vi "img_make_cam2.vi"() -> ()   [LabVIEW 2016]
uses:
  <vilib>/userdefined/High Color/IMAQdx.ctl
  <vilib>/Utility/file.llb/Write Delimited Spreadsheet (I64).vi
  <vilib>/vision/NI_Vision_Development_Module.lvlib
  <vilib>/vision/driver/NI_Vision_Acquisition_Software.lvlib
panel:
  in  "Session In":T1="cam1"
  out "Image Pixels (U8)":u8[][](array[numeric])
  in  "save":bool
  out "img_min_val":u8
  out "img_max_val":u8
  in  "Color Plane":i32(ring)=1 items=["Red", "Green", "Blue", "Hue", "Saturation", "Luminance", "Value", "Intensity"]
  out "error out":errorcluster
  out "Image_ori":T2(plugin-control)
  in  "Optional Rectangle":i32[](array[numeric])=[508, 77, 838, 531]
  in  "fname":string="lego"
  out "size_check":i32[](array[numeric])=[28, 28]
  in  "fpath_jpg":path=path "C:/Users/NB-SH-001/Documents/Python Scripts/data/img_face/01_surprise/surprise_img"
  in  "fpath_txt":path=path "C:/Users/NB-SH-001/Documents/Python Scripts/data/img_face/01_surprise/surprise_txt"
  in  "X Resolution":i32=28
  in  "Y Resolution":i32=28
  out "count":i32=91
  in  "정지":bool
  out "Image_resample":T2(plugin-control)
  # "Image file maker"
  # "28"
  # "28"
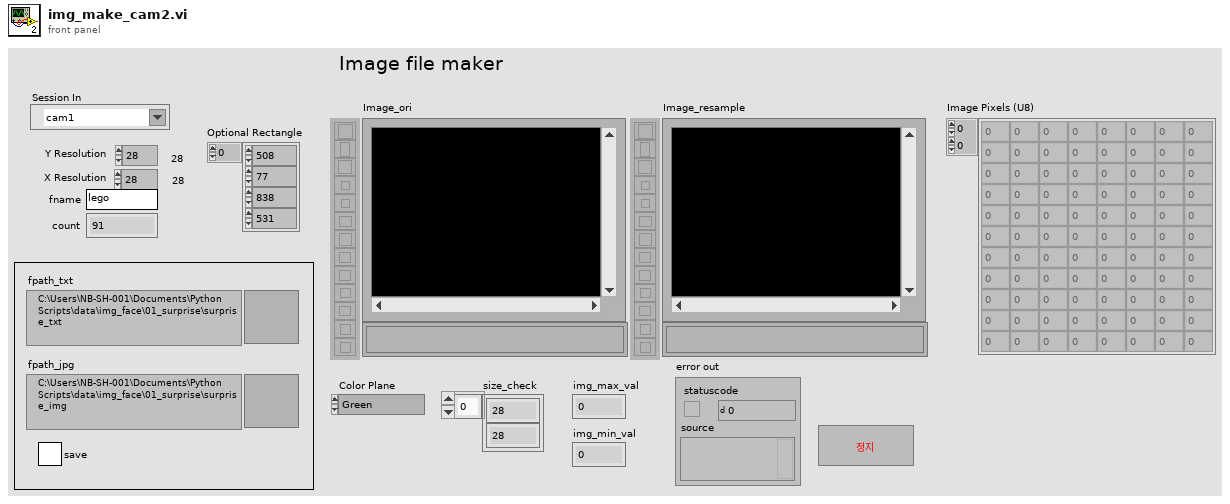
[diagram p1: front panel]
types:
  T1 = typedef "IMAQdx.ctl" = refnum<k21>
  T2 = typedef "IMAQ Image.ctl" = refnum<image>
  T3 = typedef "Image Type" = u32
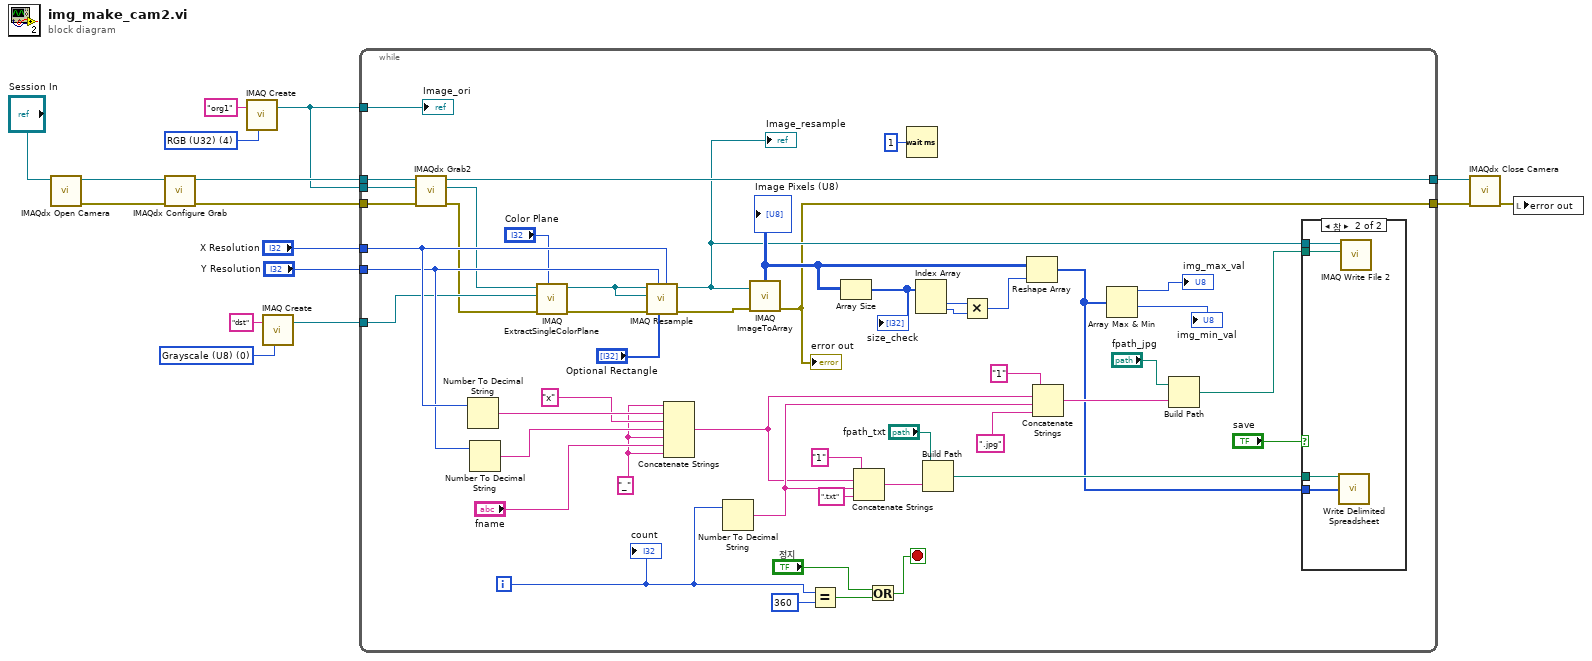
[diagram p0: block diagram]
diagram:
  w9 = T3 0 items=["Grayscale (U8)", "Grayscale (I16)", "Grayscale (SGL)", "Complex (CSG)", "RGB (U32)", "HSL (U32)", "RGB (U64)", "Grayscale (U16)"] ("Image Type")
  w15 = T3 4 items=["Grayscale (U8)", "Grayscale (I16)", "Grayscale (SGL)", "Complex (CSG)", "RGB (U32)", "HSL (U32)", "RGB (U64)", "Grayscale (U16)"] ("Image Type")
  n1 = call <vilib>:"IMAQdx Open Camera.vi"("Session In"="Session In") -> ("error out"=w11:errorcluster, "Session Out"=w12:T1)  [unwired: 9 in]
  n2 = call <vilib>:"IMAQdx Configure Grab.vi"("error in"=w11, "Session In"=w12) -> ("error out"=w7:errorcluster, "Session Out"=w6:T1)  [unwired: 8 in]
  n3 = call "IMAQ Create"("Image Name"="org1", "Image Type"=w15) -> ("New Image"=w3:T2)  [unwired: 3 in, 1 out]
  n4 = call "IMAQ Create"("Image Name"="dst", "Image Type"=w9) -> ("New Image"=w5:T2)  [unwired: 3 in, 1 out]
  n5 = while {
    tunnel: "X Resolution" -> [w34]
    tunnel: "Y Resolution" -> [w33]
    tunnel: w7 -> [w38]
    tunnel: w6 -> [w37]
    tunnel: w3 -> [w35]
    tunnel: w5 -> [w27]
    tunnel: [w32] -> w4
    tunnel: w3 -> [w29]
    tunnel: [w17] -> w2
    i -> [w57]
    stop <- w61 stop-if-true
    w40 = "_" ("문자열")
    n6 = call <vilib>:"IMAQdx Grab2.vi"("error in"=w38, "Image In"=w35, "Session In"=w37) -> ("error out"=w18:errorcluster, "Image Out"=w28:T2, "Session Out"=w32:T1)  [unwired: 5 in, 1 out]
    n7 = Number To Decimal String(number=w34) -> (decimal integer string=w44:string)  [unwired: 1 in]
    n8 = Number To Decimal String(number=w33) -> (decimal integer string=w42:string)  [unwired: 1 in]
    n9 = call "IMAQ ExtractSingleColorPlane"("Color Plane"="Color Plane", "error in (no error)"=w18, "Image Dst"=w27, "Image Src"=w28) -> ("error out"=w26:errorcluster, "Image Dst Out"=w30:T2)  [unwired: 6 in]
    n10 = call "IMAQ Resample"("X Resolution"=w34, "Optional Rectangle"="Optional Rectangle", "Y Resolution"=w33, "error in (no error)"=w26, "Image Dst"=w30, "Image Src"=w30) -> ("error out"=w22:errorcluster, "Image Dst Out"=w31:T2)  [unwired: 4 in]
    "Image_resample" <- w31
    n11 = Concatenate Strings(w40, w44, "x" ("문자열"), w42, w40, "fname", w40) -> (w39:string)
    n12 = Number To Decimal String(number=w57) -> (decimal integer string=w48:string)  [unwired: 1 in]
    n13 = call "IMAQ ImageToArray"("error in (no error)"=w22, "Image"=w31) -> ("error out"=w17:errorcluster, "Image Pixels (U8)"=w45:u8[][])  [unwired: 2 in, 3 out]
    "error out" <- w17
    "Image Pixels (U8)" <- w45
    n14 = Equal?(x=w57, y=360) -> (x = y?=w63:bool)
    n15 = Array Size(array=w45) -> (size(s)=w54:i32[])
    "size_check" <- w54
    n16 = Concatenate Strings("1" ("문자열"), w39, w48, ".txt" ("문자열")) -> (w59:string)
    n17 = Or(x="정지", y=w63) -> (x .or. y?=w61:bool)
    n18 = Wait (ms)(milliseconds to wait=u32 1 ("대기 시간 (ms)")) -> ()  [unwired: 1 out]
    n19 = Index Array(array=w54) -> (element #1=w52:i32, element #2=w53:i32)  [unwired: 2 in]
    n20 = Build Path(base path="fpath_txt", name or relative path=w59) -> (appended path=w21:path)
    n21 = Multiply(x=w52, y=w53) -> (x*y=w55:i32)
    n22 = Reshape Array(w45, w55) -> (w20:u8[])
    n23 = Concatenate Strings("1" ("문자열"), w39, w48, ".jpg" ("문자열")) -> (w50:string)
    n24 = Array Max & Min(array=w20) -> (max value=→"img_max_val":u8, min value=→"img_min_val":u8)  [unwired: 2 out]
    n25 = Build Path(base path="fpath_jpg", name or relative path=w50) -> (appended path=w46:path)
    n26 = case shown="참" "save" {
      tunnel: w46 -> [_ w69]
      tunnel: w31 -> [_ w68]
      tunnel: w21 -> [_ w67]
      tunnel: w20 -> [_ w66]
      frame False {
      }
      frame True {
        n27 = call-poly <vilib>:"Write Delimited Spreadsheet.vi"("file path (dialog if empty)"=w67, "1D data"=w66) -> ()  [unwired: 12 in, 2 out]
        n28 = call-poly "IMAQ Write File 2"("File Path"=w69, "Image"=w68) -> ()  [unwired: 8 in, 2 out]
      }
    }
    "count" <- w57
    "Image_ori" <- w29
  }
  n29 = call <vilib>:"IMAQdx Close Camera.vi"("error in"=w2, "Session In"=w4) -> ("error out"=w1:errorcluster)  [unwired: 9 in]
  n30 = local write "error out"(w1) -> ()
